vi "get Address.vi"(11 "IO in":refnum<class "IO.lvclass">) -> (3 "Address":u16 format="%04x")   [LabVIEW 2021, in "IO.lvclass"]
uses:
  IO.lvclass
  IO.lvclass/IO.ctl
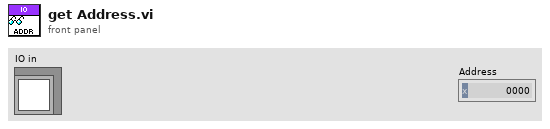
[diagram p1: front panel]
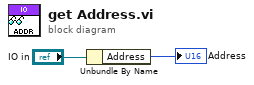
[diagram p0: block diagram]
diagram:
  n1 = Unbundle By Name("IO in") -> ("Address"=→"Address":u16)
